vi "InitializeSessions.vi"(0 "Keysight_34401A-DMM in":refnum<class "Keysight_34401A-DMM.lvclass">, 5 "InitializeSessionsInfo":variant, 11 "error in (no error)":errorcluster) -> (4 "Keysight_34401A-DMM out":refnum<class "Keysight_34401A-DMM.lvclass">, 15 "error out":errorcluster)   [LabVIEW 2020, in "Abstract_Instrument.lvlib" / "Keysight_34401A-DMM.lvclass"]
uses:
  Keysight_34401A-DMM.lvclass
  C:/Program Files/National Instruments/LabVIEW 2020/vi.lib/MeasurementLink/MeasurementLink Instrument/ISession Factory/ISession Factory.lvclass
  TypeDef/Initialize_Information.ctl
  <vilib>/MeasurementLink/MeasurementLink Session Management V1/Session Reservation/Initialize and Close Session Behavior.ctl
  Keysight_34401A-DMM.lvclass/Keysight_34401A-DMM.ctl
  b116fd11-a7c2-4259-97aa-a06ad338d6e7.vi
  <vilib>/MeasurementLink/MeasurementLink Session Management V1/Session Reservation/Initialize Sessions with Retry.vi
  <vilib>/MeasurementLink/MeasurementLink Session Management V1/Session Reservation/Session Reservation.lvclass
panel:
  out "channel list":string
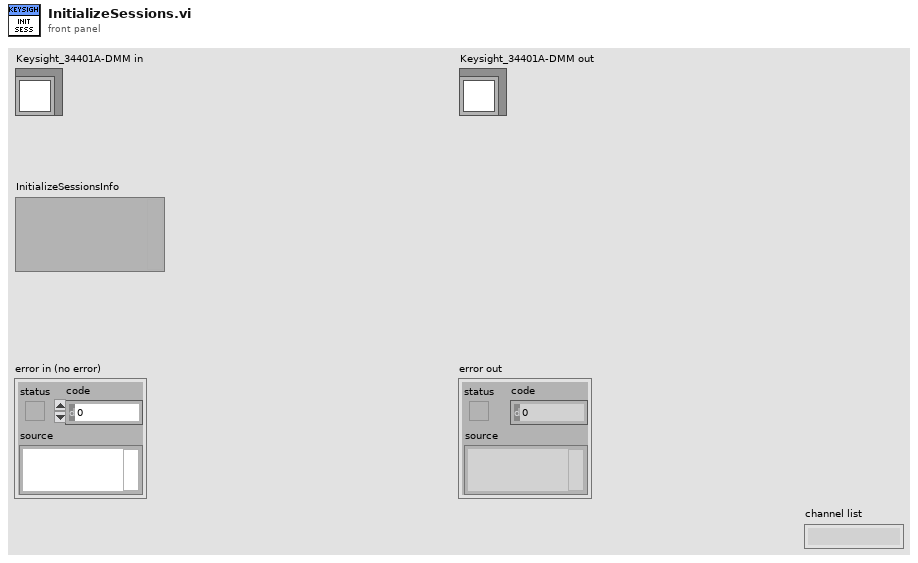
[diagram p1: front panel]
types:
  T1 = cluster{"Baud Rate":u32, "Parity":u16, "Data Bits":u16}
  T2 = typedef "Abstract_Instrument.lvlib/Keysight_34401A-DMM.lvclass/Initialize_Information.ctl" = cluster{"initialize and close session behavior":T3, "reset":bool}
  T3 = typedef "MeasurementLink Session Management V1.lvlib/Session Reservation.lvclass/Initialize and Close Session Behavior.ctl" = enum16{"Auto", "Initialize and Close", "Attach and Detach", "Initialize and Detach", "Attach and Close"}
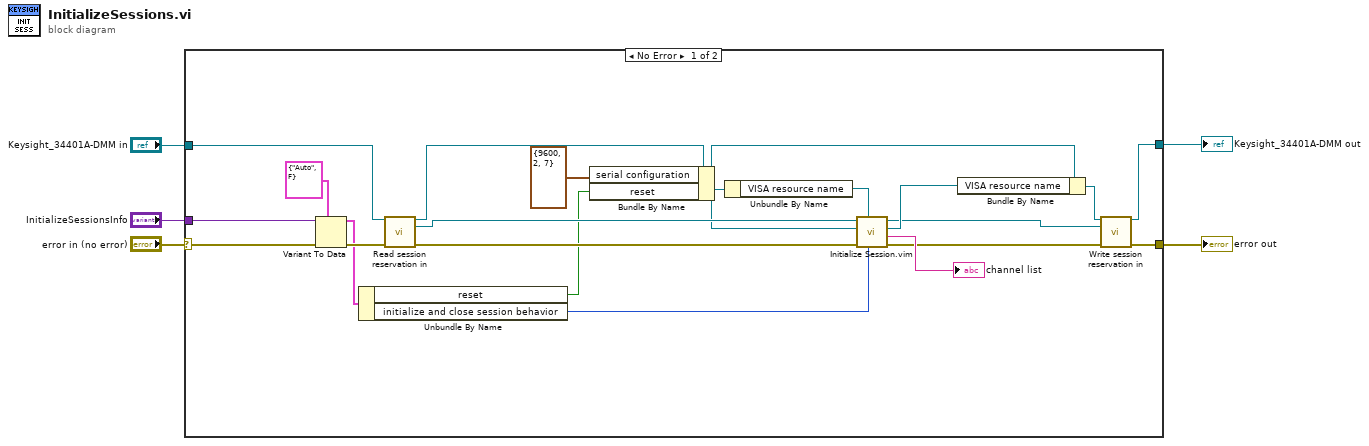
[diagram p0: block diagram]
diagram:
  n1 = case shown="No Error" "error in (no error)" {
    selector: "error in (no error)" -> [w25 w27]
    tunnel: "Keysight_34401A-DMM in" -> [w26 w28]
    tunnel: [w11 w27] -> w3
    tunnel: "InitializeSessionsInfo" -> [w23 _]
    tunnel: [w9 w28] -> w1
    frame No Error {
      n2 = Variant To Data(error in=w25, type=T2 {"initialize and close session behavior"=enum."Auto", "reset"=FALSE} ("Initialize_Information"), Variant=w23) -> (data=w21:T2, error out=w24:errorcluster)
      n3 = Unbundle By Name(w21) -> ("reset"=w14:bool, "initialize and close session behavior"=w15:T3)
      n4 = call-dynamic "Read session reservation in.vi"("AbstractDMM in"=w26, "error in (no error)"=w24) -> ("AbstractDMM out"=w22:refnum<class "Keysight_34401A-DMM.lvclass">, "MeasurementLink Session Management V1.lvlib:Session Reservation.lvclass"=w17:refnum<class "Session Reservation.lvclass">, "error out"=w18:errorcluster)  [unwired: 11 in]
      n5 = Bundle By Name(cluster=w22, "serial configuration"=T1 {"Baud Rate"=9600, "Parity"=2, "Data Bits"=7}, "reset"=w14) -> (w7:refnum<class "Keysight_34401A-DMM.lvclass">)
      n6 = Unbundle By Name(w7) -> ("VISA resource name"=w6:refnum<visa-resource-name>)
      n7 = call "Initialize Session.vim"("initialize and close session behavior"=w15, "session type"=w6, "error in"=w18, "session factory"=w7, "session reservation in"=w17) -> ("error out"=w12:errorcluster, "channel list"=→"channel list":string, "session"=w13:refnum<visa-resource-name>, "session reservation out"=w8:refnum<class "Session Reservation.lvclass">)  [unwired: 3 in]
      n8 = Bundle By Name(cluster=w7, "VISA resource name"=w13) -> (w10:refnum<class "Keysight_34401A-DMM.lvclass">)
      n9 = call-dynamic "Write session reservation in.vi"("AbstractDMM in"=w10, "MeasurementLink Session Management V1.lvlib:Session Reservation.lvclass"=w8, "error in (no error)"=w12) -> ("AbstractDMM out"=w9:refnum<class "Keysight_34401A-DMM.lvclass">, "error out"=w11:errorcluster)  [unwired: 11 in]
    }
    frame Error {
    }
  }
  "error out" <- w3
  "Keysight_34401A-DMM out" <- w1
